vi "Continuous Voltage - Left - Right - NI.vi"() -> ()   [LabVIEW 2022 SP3]
uses:
  <vilib>/DAQmx/write.llb/DAQmx Write (Analog 1D DBL 1Chan NSamp).vi
  <vilib>/DAQmx/create/channels.llb/DAQmx Create Channel (AO-Voltage-Basic).vi
  <vilib>/DAQmx/configure/timing.llb/DAQmx Timing (Sample Clock).vi
  <vilib>/DAQmx/miscellaneous.llb/DAQmx Fill In Error Info.vi
  <vilib>/measure/NI_MABase.lvlib
panel:
  out "Waveform Graph":waveform(dbl)[](graph)
  in  "Sampling Rate":i32=50000
  in  "Number of Samples":i32=50000
  in  "stop":bool
  in  "Frequency Left":dbl(slide)=10.0 scale=1.0..2000.0
  in  "Amplitude Left":dbl(slide)=1.0 scale=0.0..2.0
  in  "Frequency Right":dbl(slide)=10.0 scale=10.0..2000.0
  in  "Amplitude Right":dbl(slide)=1.0 scale=0.0..2.0
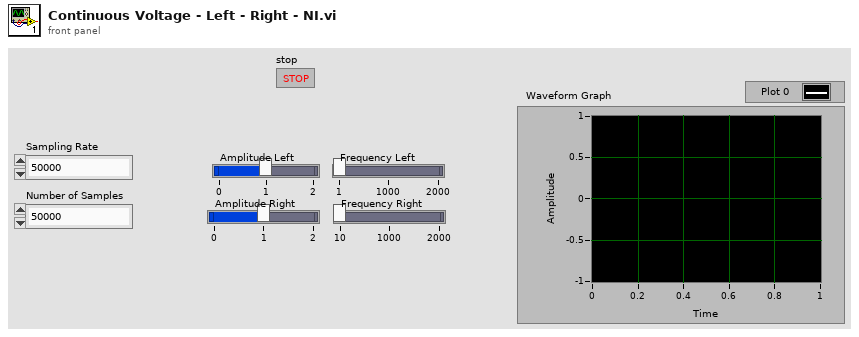
[diagram p1: front panel]
types:
  T1 = cluster{"Sampling Rate":i32, "Number of Samples":i32}
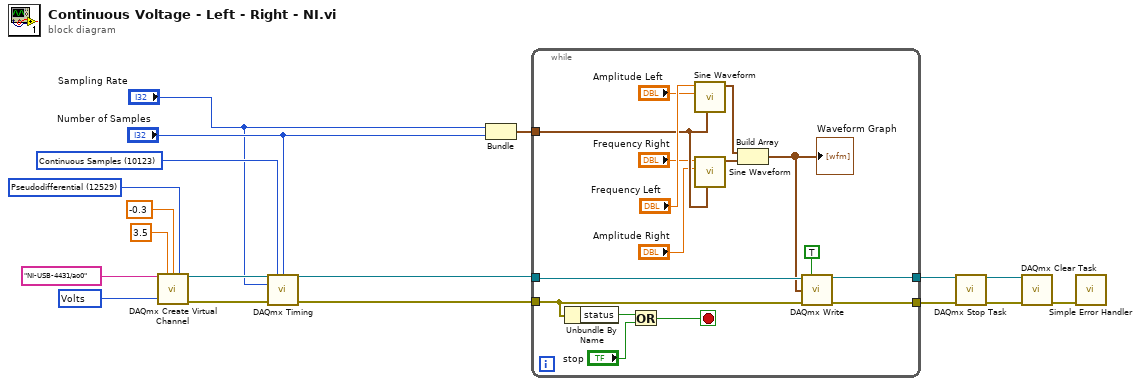
[diagram p0: block diagram]
diagram:
  w9 = 10123 items=["Finite Samples"=10178, "Continuous Samples"=10123, "Hardware Timed Single Point"=12522] ("sample mode")
  w11 = 12529 items=["Default"=-1, "RSE"=10083, "Differential"=10106, "Pseudodifferential"=12529] ("output terminal configuration")
  w13 = 10348 items=["Volts"=10348, "From Custom Scale"=10065] ("units")
  n1 = call-poly <vilib>:"DAQmx Create Virtual Channel.vi"("maximum value"=3.5, "minimum value"=-0.3, "output terminal configuration"=w11, "physical channels"=tag "NI-USB-4431/ao0", "units"=w13) -> ("task out"=w16:refnum<k21>, "error out"=w17:errorcluster)  [unwired: 9 in]
  n2 = call-poly <vilib>:"DAQmx Timing.vi"("task/channels in"=w16, "sample mode"=w9, "samples per channel"="Number of Samples", "rate"="Sampling Rate", "error in"=w17) -> ("task out"=w2:refnum<k21>, "error out"=w1:errorcluster)  [unwired: 9 in]
  n3 = Bundle("Sampling Rate"="Sampling Rate", "Number of Samples"="Number of Samples") -> (w18:T1)  [unwired: 1 in]
  n4 = while {
    tunnel: w2 -> [w24]
    tunnel: w1 -> [w23]
    tunnel: w18 -> [w27]
    tunnel: [w22] -> w7
    tunnel: [w21] -> w6
    stop <- w32 stop-if-true
    n5 = Unbundle By Name(w23) -> ("status"=w30:bool)
    n6 = Or(x=w30, y="stop") -> (x .or. y?=w32:bool)
    n7 = call <vilib>:"Sine Waveform.vi"("sampling info"=w27, "amplitude"="Amplitude Left", "frequency"="Frequency Left") -> ("signal out"=w29:waveform(dbl))  [unwired: 7 in, 1 out]
    n8 = call <vilib>:"Sine Waveform.vi"("sampling info"=w27, "amplitude"="Amplitude Right", "frequency"="Frequency Right") -> ("signal out"=w28:waveform(dbl))  [unwired: 7 in, 1 out]
    n9 = Build Array(w29, w28) -> (w20:waveform(dbl)[])
    "Waveform Graph" <- w20
    n10 = call-poly <vilib>:"DAQmx Write.vi"("task/channels in"=w24, "auto start"=TRUE, "data"=w20, "error in"=w23) -> ("task out"=w21:refnum<k21>, "error out"=w22:errorcluster)  [unwired: 9 in, 1 out]
  }
  n11 = call <vilib>:"DAQmx Stop Task.vi"("task/channels in"=w6, "error in"=w7) -> ("task out"=w4:refnum<k21>, "error out"=w5:errorcluster)  [unwired: 12 in]
  n12 = call <vilib>:"DAQmx Clear Task.vi"("task in"=w4, "error in"=w5) -> ("error out"=w3:errorcluster)  [unwired: 13 in]
  n13 = call <vilib>:"Simple Error Handler.vi"("error in (no error)"=w3) -> ()  [unwired: 4 in, 5 out]
